vi "Write Tab Layout.vi"(5 "Tab Layout":T1(ring), 9 "Tab in":refnum<class "Tab.lvclass">) -> (3 "Tab out":refnum<class "Tab.lvclass">)   [LabVIEW 2014, in "Tab.lvclass"]
uses:
  Tab.lvclass
  Tab.lvclass/Tab.ctl
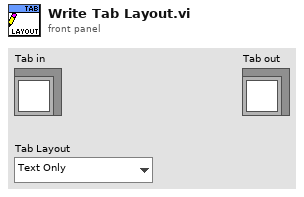
[diagram p1: front panel]
types:
  T1 = enum32{"Text Only", "Image Only", "Text - Image", "Image - Text"}
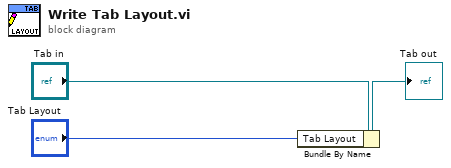
[diagram p0: block diagram]
diagram:
  n1 = Bundle By Name(cluster="Tab in", "Tab Layout"="Tab Layout") -> (→"Tab out":refnum<class "Tab.lvclass">)
